vi "Rename Channel.vi"(7 "Channels Ctrl Ref":refnum<vi>, 8 "error in (no error)":errorcluster, 11 "To Save Wfm Arrays":waveform(dbl)[](array[waveform])) -> (0 "error out":errorcluster, 2 "Udpated Wfm Grp Data":T1, 3 "Channel Renamed?":bool)   [LabVIEW 2025, in "TDMS Waveform Creator UI.lvlib"]
uses:
  TDMS Waveform Creator UI.lvlib
panel:
  in  "Cancel":bool
  in  "OK":bool
  in  "Channel Name":string
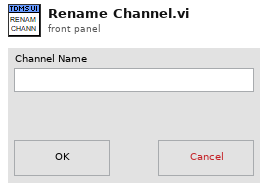
[diagram p1: front panel]
types:
  T1 = cluster{"Channel Names":string[], "To Save Wfm Arrays":waveform(dbl)[], "Waveform Summary JSON":string[]}
  T2 = cluster{"Item Names":string[], waveform(dbl)[], string[]}
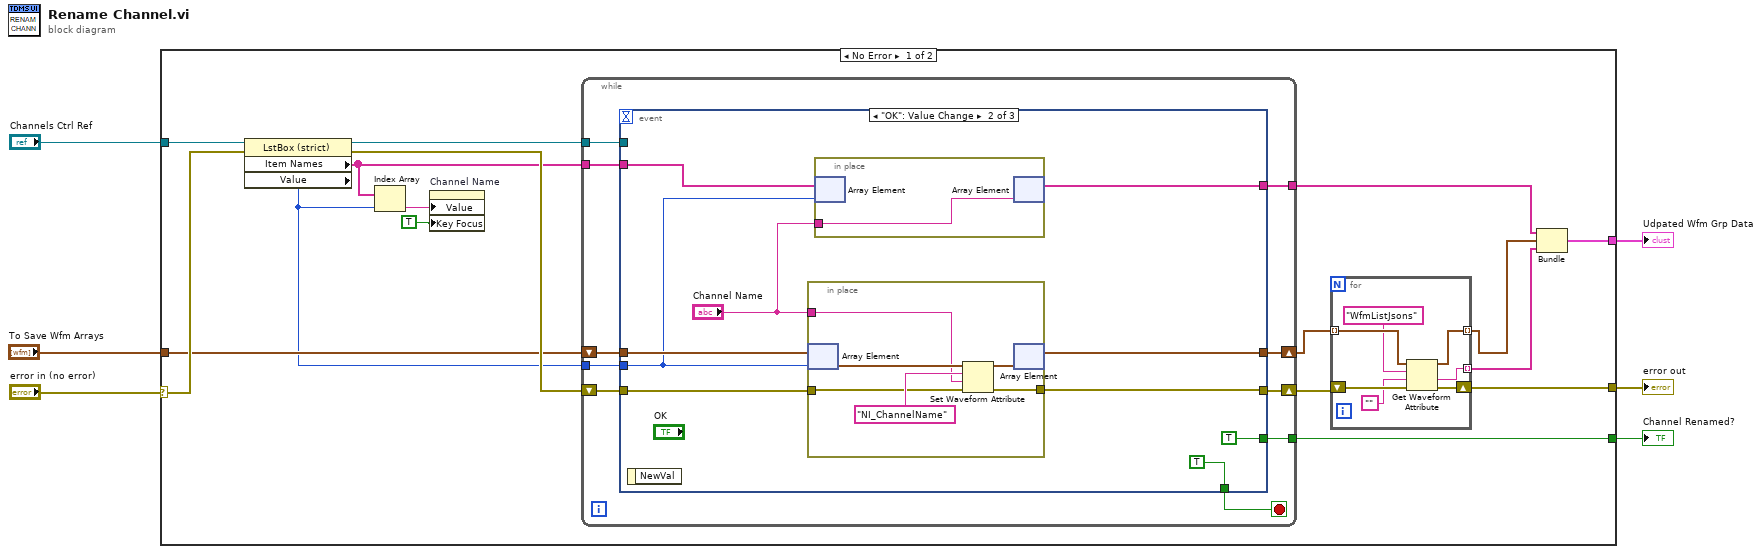
[diagram p0: block diagram]
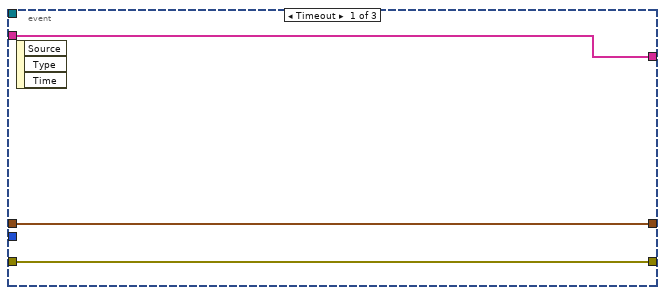
[diagram p2: hidden frame]
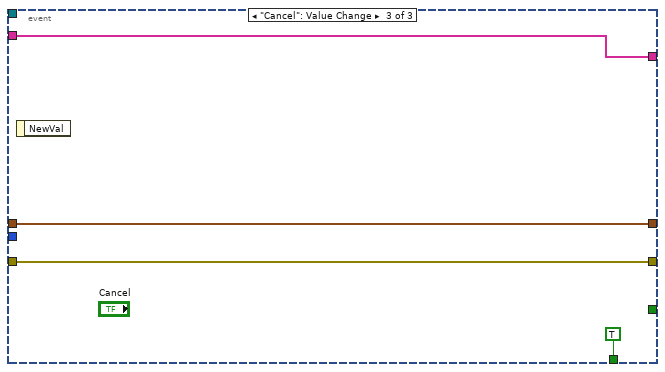
[diagram p3: hidden frame]
diagram:
  n1 = case shown="No Error" "error in (no error)" {
    selector: "error in (no error)" -> [w21 w65]
    tunnel: "Channels Ctrl Ref" -> [w23 _]
    tunnel: "To Save Wfm Arrays" -> [w18 _]
    tunnel: [w13 w65] -> w3
    tunnel: [w15 _] -> w2
    tunnel: [w8 _] -> w1
    frame No Error {
      n2 = property class="LstBox (strict)"(reference=w23, error in=w21) -> (reference out=w22:refnum<vi>, error out=w20:errorcluster, "Item Names"=w16:string[], "Value"=w17:i32)
      n3 = Index Array(array=w16, index=w17) -> (element=w19:string)
      n4 = property on="Channel Name" class="Str"("Value"=w19, "Key Focus"=TRUE) -> ()  [unwired: 2 in, 2 out]
      n5 = while {
        tunnel: w22 -> [w40]
        tunnel: w17 -> [w36]
        tunnel: w16 -> [w35]
        shift-right: [w38] -> w12
        shift-left: w20 -> [w39]
        shift-right: [w34] -> w14
        shift-left: w18 -> [w37]
        tunnel: [w32] -> w15
        tunnel: [w31] -> w11
        stop <- w33 stop-if-true
        n6 = event shown="[1] \"OK\": Value Change" {
          selector: _ -> [_ _ _]
          dyn-events: _ -> [_ _ _]
          timeout: _ -> [_ _ _]
          tunnel: w40 -> [_ _ _]
          tunnel: w39 -> [w42 w53 w62]
          tunnel: [w42 w52 w62] -> w38
          tunnel: w37 -> [w41 w51 w61]
          tunnel: w36 -> [_ w46 _]
          tunnel: w35 -> [w43 w50 w63]
          tunnel: [w41 w48 w61] -> w34
          tunnel: [_ TRUE TRUE] -> w33
          tunnel: [_ TRUE _] -> w32
          tunnel: [w43 w44 w63] -> w31
          event Timeout {
            n7 = event-data() -> ()  [unwired: 1 in, 3 out]
          }
          event "OK": Value Change {
            n8 = event-data() -> ()  [unwired: 1 in, 1 out]
            n9 = in-place {
              in-place-border: w53 -> [w59]
              in-place-border: [w58] -> w52
              in-place-border: "Channel Name" -> [w56]
              n10 = in-place-array #1(w51, w46) -> (w57:waveform(dbl))
              n11 = Set Waveform Attribute(4:w59, 5:w56, 6:"NI_ChannelName" ("name"), 7:w57) -> (0:w58:errorcluster, 3:w55:waveform(dbl))  [unwired: 1 out]
              n12 = in-place-array #1(w55) -> (w48:waveform(dbl)[])  [unwired: 1 out]
            }
            n13 = in-place {
              in-place-border: "Channel Name" -> [w54]
              n14 = in-place-array #2(w50, w46) -> ()  [unwired: 1 out]
              n15 = in-place-array #2(w54) -> (w44:string[])  [unwired: 1 out]
            }
          }
          event "Cancel": Value Change {
            n16 = event-data() -> ()  [unwired: 1 in, 1 out]
          }
        }
      }
      n17 = for {
        shift-right: [w29] -> w13
        shift-left: w12 -> [w30]
        tunnel: w14 -> [w28] mode=indexing
        tunnel: [w27] -> w10 mode=indexing
        tunnel: [w24] -> w9 mode=indexing
        n18 = Get Waveform Attribute(4:w30, 5:"", 6:"WfmListJsons" ("name"), 7:w28) -> (0:w29:errorcluster, 1:w24:string, 3:w27:waveform(dbl))  [unwired: 1 out]
      }
      n19 = Bundle("Item Names"=w11, w10, w9) -> (w8:T2)  [unwired: 1 in]
    }
    frame Error {
    }
  }
  "error out" <- w3
  "Channel Renamed?" <- w2
  "Udpated Wfm Grp Data" <- w1
